vi "LWXPS_MultipleAxesPVTPulseOutputGet.vi"(0 "XPS Reference IN":refnum<k24>, 5 "Group Name":string, 11 "LabVIEW error IN":errorcluster) -> (3 "XPS Reference OUT":refnum<k24>, 4 "Returned error code":i32, 6 "Start Element":i32, 8 "End Element":i32, 10 "Time Interval":dbl, 14 "LabVIEW error OUT":errorcluster, 15 "XPS Error String":string)   [LabVIEW 2014]
uses:
  D:/XPSQ8_LabView_Library/Development/Source/Dll/Newport.XPS.CommandInterface.dll
  Dll/Newport.XPS.CommandInterface.dll
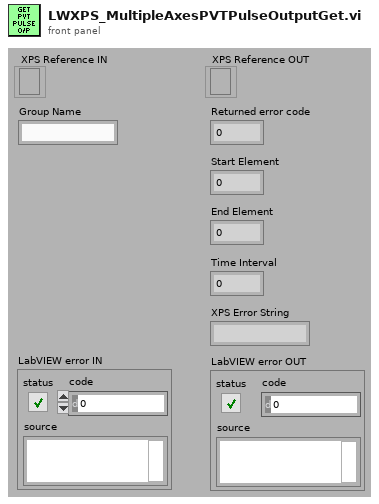
[diagram p1: front panel]
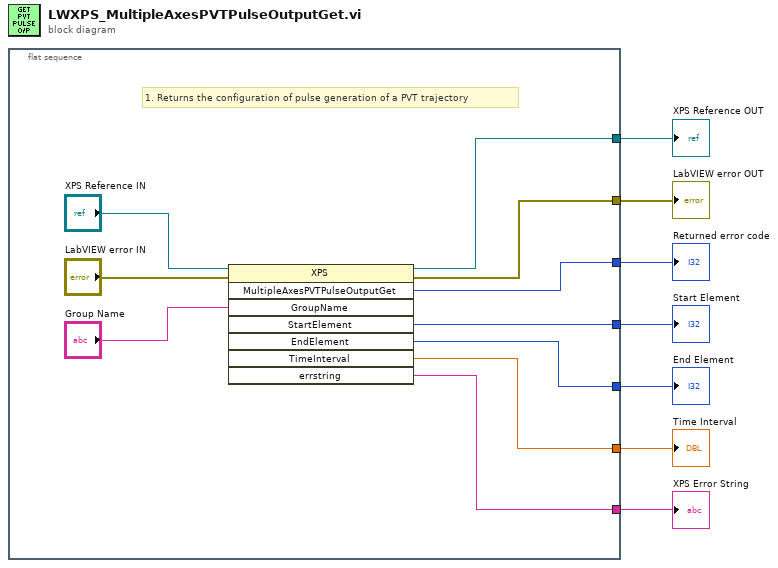
[diagram p0: block diagram]
diagram:
  n1 = flat-sequence {
    tunnel: [w15] -> w7
    tunnel: [w17] -> w6
    tunnel: [w14] -> w5
    tunnel: [w11] -> w2
    tunnel: [w10] -> w3
    tunnel: [w9] -> w1
    tunnel: [w8] -> w4
    frame #0 {
      # "1. Returns the configuration of pulse generation of a PVT trajectory"
      n2 = invoke class="XPS" method="MultipleAxesPVTPulseOutputGet"(reference="XPS Reference IN", error in="LabVIEW error IN", "GroupName"="Group Name") -> (reference out=w15:refnum<k24>, error out=w17:errorcluster, "MultipleAxesPVTPulseOutputGet"=w14:i32, "StartElement"=w10:i32, "EndElement"=w11:i32, "TimeInterval"=w9:dbl, "errstring"=w8:string)  [unwired: 5 in, 1 out]
    }
  }
  "XPS Reference OUT" <- w7
  "LabVIEW error OUT" <- w6
  "Returned error code" <- w5
  "XPS Error String" <- w4
  "Start Element" <- w3
  "End Element" <- w2
  "Time Interval" <- w1
